vi "Apply_Flips_2_Coords.vi"(9 "Max Array":i32[](array[numeric]), 10 "Coords in":cluster{"X":i32, "Y":i32}[](array[cluster]), 11 "Draw_ops":T1) -> (2 "Coords out":cluster{"X":i32, "Y":i32}[](array[cluster]))   [LabVIEW 2010]
doc: "This VI is used to flip the set of coordinates vertically and horizontally if desired.\n\nCreated by Davis Montenegro\n20-06-2016"
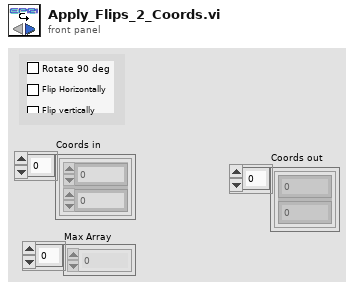
[diagram p1: front panel]
types:
  T1 = cluster{"Rotate 90 deg":bool, "Flip Horizontally":bool, "Flip vertically":bool}
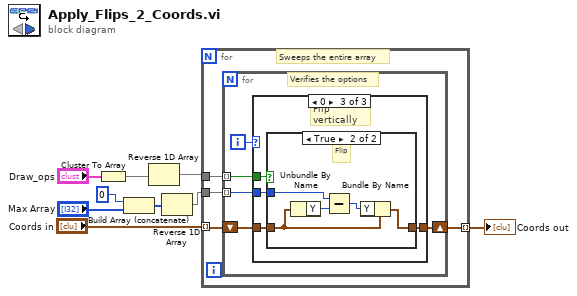
[diagram p0: block diagram]
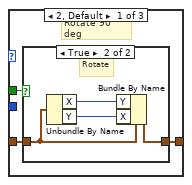
[diagram p2: hidden frame]
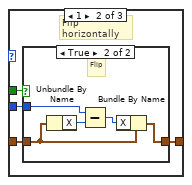
[diagram p4: hidden frame]
diagram:
  n1 = Cluster To Array(cluster="Draw_ops") -> (array=w4:bool[])
  n2 = Build Array (concatenate)(0 ("Max Y"), "Max Array") -> (w2:i32[])
  n3 = Reverse 1D Array(array=w4) -> (reversed array=w3:bool[])
  n4 = Reverse 1D Array(array=w2) -> (reversed array=w1:i32[])
  n5 = for {
    tunnel: w1 -> [w13]
    tunnel: w3 -> [w12]
    tunnel: "Coords in" -> [w11] mode=indexing
    tunnel: [w10] -> w7 mode=indexing
    # "Sweeps the entire array"
    n6 = for {
      tunnel: w12 -> [w17] mode=indexing
      tunnel: w13 -> [w15] mode=indexing
      shift-right: [w14] -> w10
      shift-left: w11 -> [w16]
      i -> [w18]
      # "Verifies the options"
      n7 = case shown="0" w18 {
        tunnel: w17 -> [w21 w30 w40]
        tunnel: w16 -> [w20 w28 w38]
        tunnel: w15 -> [_ w29 w39]
        tunnel: [w19 w27 w37] -> w14
        frame 2, Default {
          # "Rotate 90 deg"
          n8 = case shown="True" w21 {
            tunnel: w20 -> [w22 w26]
            tunnel: [w22 w25] -> w19
            frame False {
              # "Keep it the same"
            }
            frame True {
              # "Rotate"
              n9 = Unbundle By Name(w26) -> ("X"=w23:i32, "Y"=w24:i32)
              n10 = Bundle By Name(cluster=w26, "Y"=w23, "X"=w24) -> (w25:cluster{"X":i32, "Y":i32})
            }
          }
        }
        frame 1 {
          # "Flip horizontally"
          n11 = case shown="True" w30 {
            tunnel: w29 -> [_ w32]
            tunnel: w28 -> [w31 w36]
            tunnel: [w31 w35] -> w27
            frame False {
              # "No Flip"
            }
            frame True {
              # "Flip"
              n12 = Unbundle By Name(w36) -> ("X"=w34:i32)
              n13 = Subtract(x=w32, y=w34) -> (x-y=w33:i32)
              n14 = Bundle By Name(cluster=w36, "X"=w33) -> (w35:cluster{"X":i32, "Y":i32})
            }
          }
        }
        frame 0 {
          # "Flip vertically"
          n15 = case shown="True" w40 {
            tunnel: w39 -> [_ w42]
            tunnel: w38 -> [w41 w46]
            tunnel: [w41 w45] -> w37
            frame False {
              # "No Flip"
            }
            frame True {
              # "Flip"
              n16 = Unbundle By Name(w46) -> ("Y"=w44:i32)
              n17 = Subtract(x=w42, y=w44) -> (x-y=w43:i32)
              n18 = Bundle By Name(cluster=w46, "Y"=w43) -> (w45:cluster{"X":i32, "Y":i32})
            }
          }
        }
      }
    }
  }
  "Coords out" <- w7
